vi "ErrorDuringStartup.vi"(8 "error in":errorcluster) -> (0 "error out":errorcluster, 3 "Error During Startup":bool)   [LabVIEW 2020]
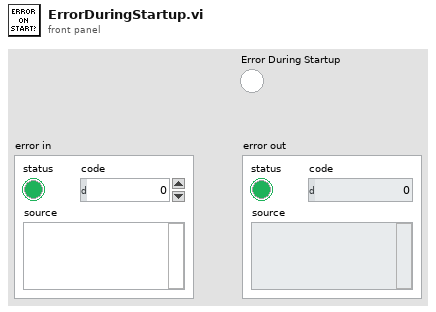
[diagram p1: front panel]
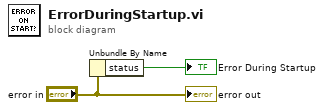
[diagram p0: block diagram]
diagram:
  n1 = Unbundle By Name("error in") -> ("status"=→"Error During Startup":bool)
  "error out" <- "error in"
